vi "Find Event Channels.vi"(6 "duration multiplier":dbl, 7 "Custom Device Ref":T1 format="%.0x", 8 "error in (no error)":errorcluster, 9 "Channel Descriptors in":T2, 11 "Event ref":T1 format="%.0x") -> (0 "error out":errorcluster, 1 "Channel Descriptors out":T2)   [LabVIEW 2011, in "Engine Sim System Explorer.lvlib"]
uses:
  Engine Sim System Explorer.lvlib
  <vilib>/NI Veristand/Custom Device API/Custom Device Item Ref.ctl
  Shared/Channel Descriptors.ctl
  Shared/FPGA Write Descriptor.ctl
  Shared/InputChannelTypes.ctl
  <vilib>/rvi/DataTransferAndStorage/Container/Common/niFpgaDataTypeControl.ctl
  Shared/FPGA Read Descriptor.ctl
  Shared/OutputChannelTypes.ctl
  Shared/Status Chan Descriptor.ctl
  Shared/Engine Simulation Global.vi
  <vilib>/NI Veristand/Custom Device Tools/Custom Device Utility Library/NI VeriStand - Search for Item by Name.vi
  <vilib>/NI Veristand/Custom Device Tools/Custom Device Utility Library/Custom Device Utility Library.lvlib
  Engine Simulation Shared.lvlib
  <vilib>/NI Veristand/Custom Device API/Custom Device API.lvlib
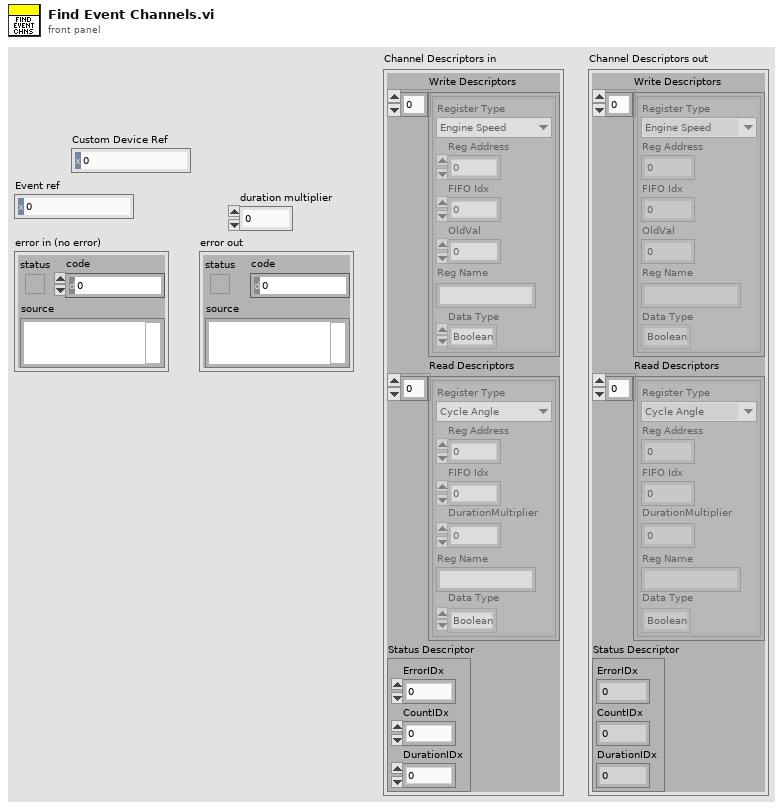
[diagram p1: front panel]
types:
  T1 = typedef "Custom Device API.lvlib/Custom Device Item Ref.ctl" = u64
  T2 = typedef "Engine Simulation Shared.lvlib/Channel Descriptors.ctl" = cluster{"Write Descriptors":T3[], "Read Descriptors":T6[], "Status Descriptor":T8}
  T3 = typedef "Engine Simulation Shared.lvlib/FPGA Write Descriptor.ctl" = cluster{"Register Type":T4, "Reg Address":u32, "FIFO Idx":i32, "OldVal":dbl, "Reg Name":string, "Data Type":T5}
  T4 = typedef "Engine Simulation Shared.lvlib/InputChannelTypes.ctl" = enum16{"Engine Speed", "Offset"}
  T5 = typedef "niFpgaDataTypeControl.ctl" = enum32{"Boolean", "I8", "I16", "I32", "I64", "U8", "U16", "U32", "U64", "FXP", "CustomControl"}
  T6 = typedef "Engine Simulation Shared.lvlib/FPGA Read Descriptor.ctl" = cluster{"Register Type":T7, "Reg Address":u32, "FIFO Idx":i32, "DurationMultiplier":dbl, "Reg Name":string, "Data Type":T5}
  T7 = typedef "Engine Simulation Shared.lvlib/OutputChannelTypes.ctl" = enum16{"Cycle Angle", "Crank Angle", "Time Duration", "Angle Duration", "Start Angle", "End Angle"}
  T8 = typedef "Engine Simulation Shared.lvlib/Status Chan Descriptor.ctl" = cluster{"ErrorIDx":i32, "CountIDx":i32, "DurationIDx":i32}
  T9 = typedef "Custom Device API.lvlib/Custom Device Item Info.ctl" = cluster{"Name":string, "Is Channel":bool, "GUID":string}
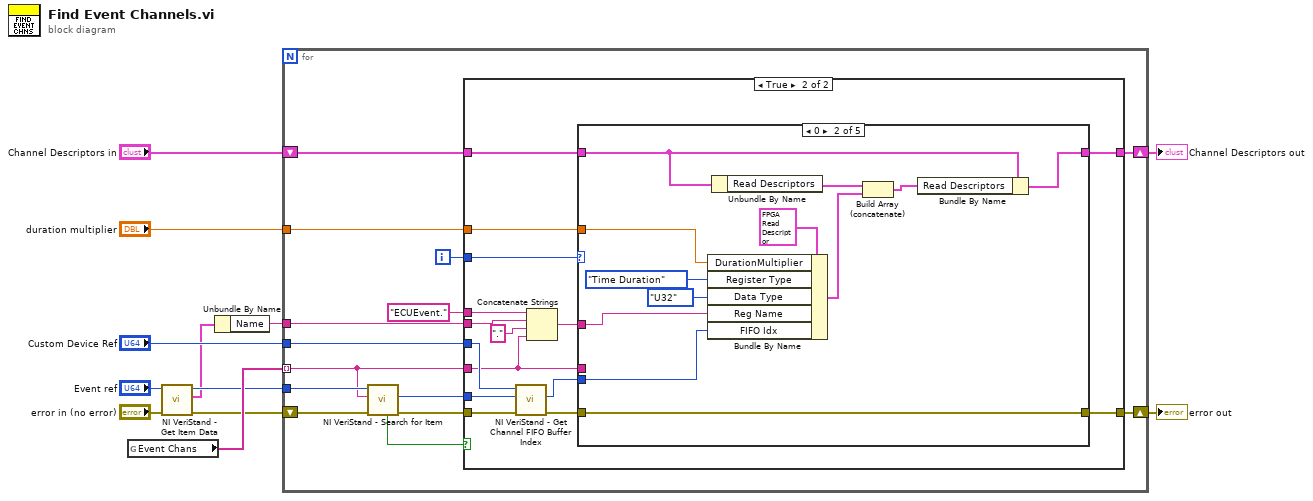
[diagram p0: block diagram]
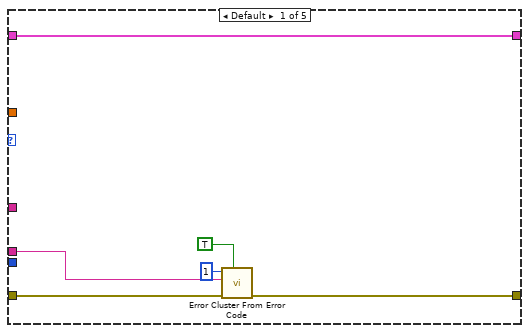
[diagram p3: hidden frame]
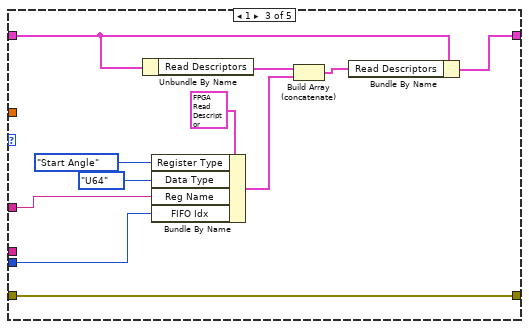
[diagram p4: hidden frame]
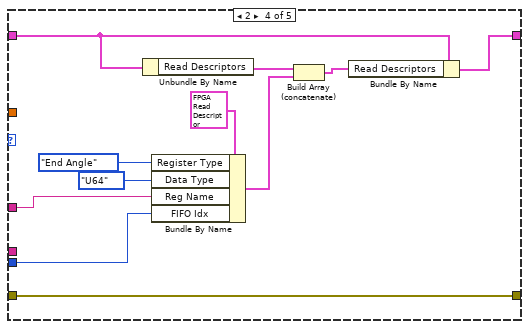
[diagram p5: hidden frame]
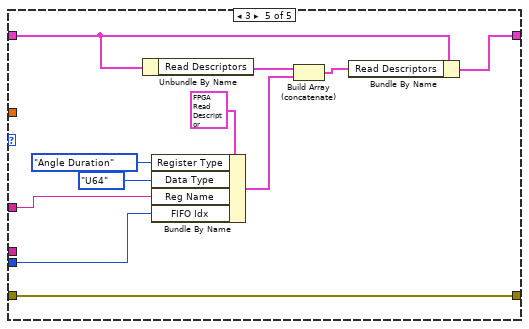
[diagram p6: hidden frame]
diagram:
  n1 = global read "Engine Simulation Global.vi" "Event Chans"() -> (w7:string[])
  n2 = call <vilib>:"NI VeriStand - Get Item Data.vi"("error in (no error)"="error in (no error)", "Item Ref in"="Event ref") -> ("error out"=w6:errorcluster, "Item Info"=w3:T9, "Item Ref out"=w4:T1)  [unwired: 6 in, 1 out]
  n3 = Unbundle By Name(w3) -> ("Name"=w2:string)
  n4 = for {
    tunnel: w4 -> [w26]
    tunnel: "Custom Device Ref" -> [w19]
    shift-right: [w16] -> w8
    shift-left: w6 -> [w25]
    shift-right: [w18] -> w9
    shift-left: "Channel Descriptors in" -> [w20]
    tunnel: w7 -> [w17] mode=indexing
    tunnel: w2 -> [w14]
    tunnel: "duration multiplier" -> [w13]
    i -> [w15]
    n5 = call-poly <vilib>:"NI VeriStand - Search for Item.vi"("error in"=w25, "Item Name"=w17, "Section Ref in"=w26) -> ("error out"=w23:errorcluster, "Item Ref"=w22:T1, "Found"=w24:bool)  [unwired: 5 in, 1 out]
    n6 = case shown="True" w24 {
      tunnel: w23 -> [w27 w42]
      tunnel: w22 -> [_ w41]
      tunnel: "ECUEvent." ("Base path") -> [_ w36]
      tunnel: w17 -> [_ w29]
      tunnel: w20 -> [w28 w43]
      tunnel: w19 -> [_ w40]
      tunnel: [w27 w30] -> w16
      tunnel: [w28 w38] -> w18
      tunnel: w15 -> [_ w37]
      tunnel: w14 -> [_ w35]
      tunnel: w13 -> [_ w32]
      frame False {
      }
      frame True {
        n7 = call <vilib>:"NI VeriStand - Get Channel FIFO Buffer Index.vi"("error in"=w42, "Channel Ref"=w41, "Device Ref in"=w40) -> ("error out"=w31:errorcluster, "Channel FIFO Buffer Index"=w39:i32)  [unwired: 4 in, 3 out]
        n8 = Concatenate Strings(w36, w35, "." ("string"), w29) -> (w33:string)
        n9 = case shown="0" w37 {
          tunnel: w43 -> [w49 w60 w71 w82 w93]
          tunnel: w39 -> [_ w58 w69 w80 w91]
          tunnel: [w49 w56 w67 w78 w89] -> w38
          tunnel: w33 -> [_ w53 w64 w75 w86]
          tunnel: w32 -> [_ w51 _ _ _]
          tunnel: w31 -> [w48 w50 w62 w73 w84]
          tunnel: [w47 w50 w62 w73 w84] -> w30
          tunnel: w29 -> [w46 _ _ _ _]
          frame Default {
            n10 = call <vilib>:"Error Cluster From Error Code.vi"("show call chain? (False)"=TRUE, "error in (no error)"=w48, "error message (\"\")"=w46, "error code (0)"=1) -> ("error out"=w47:errorcluster)  [unwired: 5 in]
          }
          frame 0 {
            n11 = Bundle By Name(cluster=T6 {"Register Type"=enum."Cycle Angle", "Reg Address"=0, "FIFO Idx"=0, "DurationMultiplier"=0.0, "Reg Name"="", "Data Type"=enum."Boolean"} ("Read Descriptor"), "DurationMultiplier"=w51, "Register Type"=OutputChannelTypes."Time Duration", "Data Type"=niFpgaDataTypeControl."U32", "Reg Name"=w53, "FIFO Idx"=w58) -> (w55:T6)
            n12 = Unbundle By Name(w60) -> ("Read Descriptors"=w61:T6[])
            n13 = Build Array (concatenate)(w61, w55) -> (w57:T6[])
            n14 = Bundle By Name(cluster=w60, "Read Descriptors"=w57) -> (w56:T2)
          }
          frame 1 {
            n15 = Unbundle By Name(w71) -> ("Read Descriptors"=w72:T6[])
            n16 = Bundle By Name(cluster=T6 {"Register Type"=enum."Cycle Angle", "Reg Address"=0, "FIFO Idx"=0, "DurationMultiplier"=0.0, "Reg Name"="", "Data Type"=enum."Boolean"} ("Read Descriptor"), "Register Type"=OutputChannelTypes."Start Angle", "Data Type"=niFpgaDataTypeControl."U64", "Reg Name"=w64, "FIFO Idx"=w69) -> (w66:T6)
            n17 = Build Array (concatenate)(w72, w66) -> (w68:T6[])
            n18 = Bundle By Name(cluster=w71, "Read Descriptors"=w68) -> (w67:T2)
          }
          frame 2 {
            n19 = Unbundle By Name(w82) -> ("Read Descriptors"=w83:T6[])
            n20 = Bundle By Name(cluster=T6 {"Register Type"=enum."Cycle Angle", "Reg Address"=0, "FIFO Idx"=0, "DurationMultiplier"=0.0, "Reg Name"="", "Data Type"=enum."Boolean"} ("Read Descriptor"), "Register Type"=OutputChannelTypes."End Angle", "Data Type"=niFpgaDataTypeControl."U64", "Reg Name"=w75, "FIFO Idx"=w80) -> (w77:T6)
            n21 = Build Array (concatenate)(w83, w77) -> (w79:T6[])
            n22 = Bundle By Name(cluster=w82, "Read Descriptors"=w79) -> (w78:T2)
          }
          frame 3 {
            n23 = Unbundle By Name(w93) -> ("Read Descriptors"=w94:T6[])
            n24 = Bundle By Name(cluster=T6 {"Register Type"=enum."Cycle Angle", "Reg Address"=0, "FIFO Idx"=0, "DurationMultiplier"=0.0, "Reg Name"="", "Data Type"=enum."Boolean"} ("Read Descriptor"), "Register Type"=OutputChannelTypes."Angle Duration", "Data Type"=niFpgaDataTypeControl."U64", "Reg Name"=w86, "FIFO Idx"=w91) -> (w88:T6)
            n25 = Build Array (concatenate)(w94, w88) -> (w90:T6[])
            n26 = Bundle By Name(cluster=w93, "Read Descriptors"=w90) -> (w89:T2)
          }
        }
      }
    }
  }
  "error out" <- w8
  "Channel Descriptors out" <- w9
